vi "2.6. форма ошибки.vi"(11 "Описание ошибки":string) -> ()   [LabVIEW 2016, in "Library.lvlib"]
uses:
  Granule-2000AT/PC/Library.lvlib
panel:
  in  "stop":bool
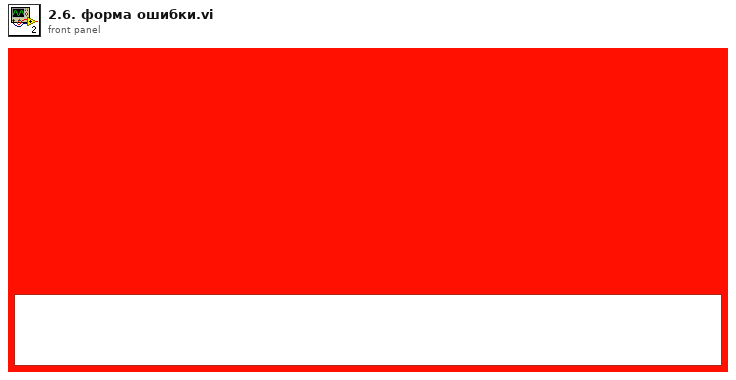
[diagram p1: front panel]
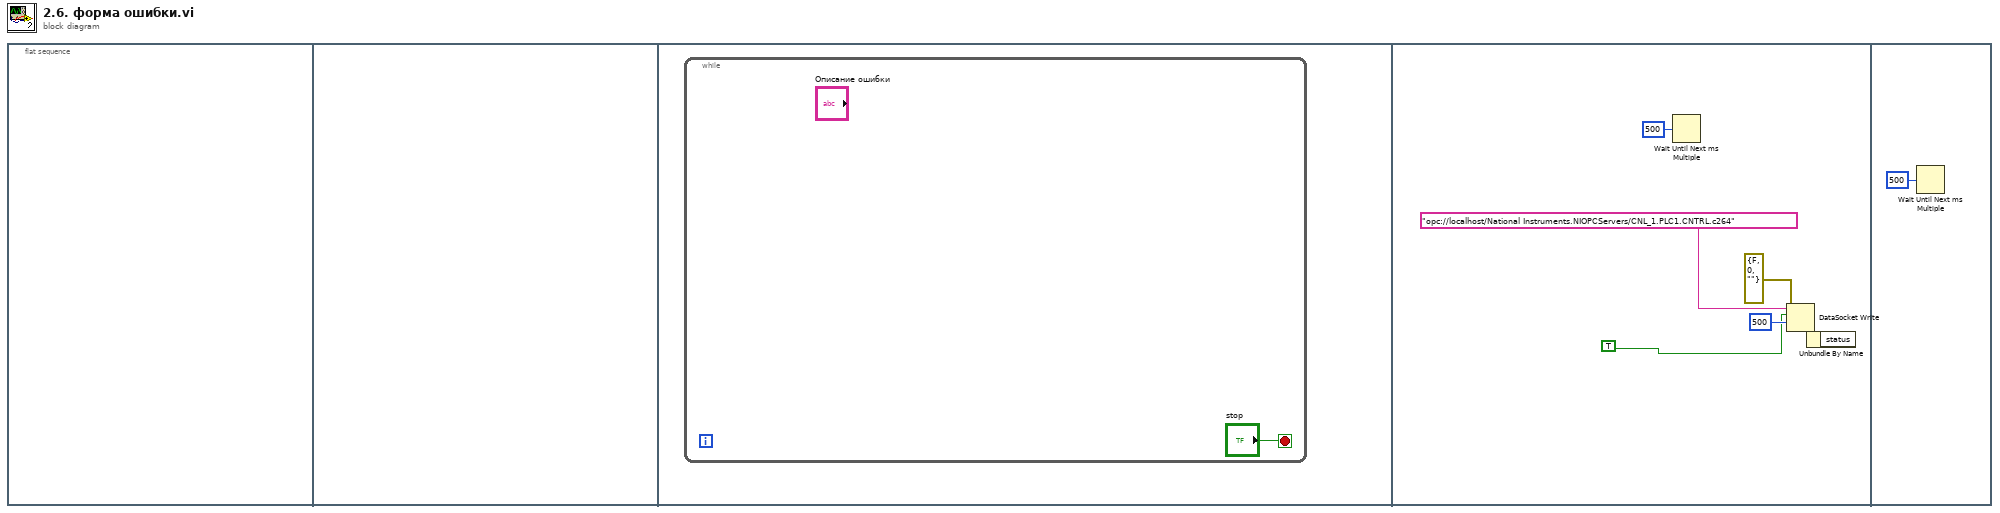
[diagram p0: block diagram]
diagram:
  n1 = flat-sequence {
    frame #0 {
    }
    frame #1 {
    }
    frame #2 {
      n2 = while {
        stop <- "stop" stop-if-true
      }
    }
    frame #3 {
      n3 = Wait Until Next ms Multiple(millisecond multiple=u32 500) -> ()  [unwired: 1 out]
      n4 = DataSocket Write(8:errorcluster {"status"=FALSE, "code"=0, "source"=""} ("error in (no error)"), 9:500 ("ms timeout (0)"), 10:TRUE, 11:"opc://localhost/National Instruments.NIOPCServers/CNL_1.PLC1.CNTRL.c264" ("connection in")) -> (0:w5:errorcluster)  [unwired: 2 out]
      n5 = Unbundle By Name(w5) -> ()  [unwired: 1 out]
    }
    frame #4 {
      n6 = Wait Until Next ms Multiple(millisecond multiple=u32 500) -> ()  [unwired: 1 out]
    }
  }
